vi "Global_CMD to Gear.vi"() -> ()   [LabVIEW 2017]
panel:
  in  "Gear wait till pullback (seconds)":dbl
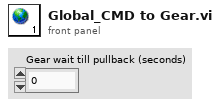
[diagram p1: front panel]
diagram:
